vi "Log Pump.vi"(1 "Log File Cluster":T1, 2 "Pumps power":dbl(slide) scale=0.0..100.0 scale format="%#_g%%") -> ()   [LabVIEW 2016]
uses:
  Log File Cluster.ctl
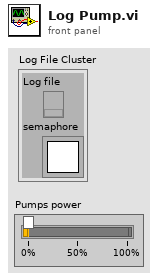
[diagram p1: front panel]
types:
  T1 = typedef "Log File Cluster.ctl" = cluster{"Log file":refnum<k34>, "semaphore":T2}
  T2 = typedef "Semaphore RefNum" = refnum<k1>
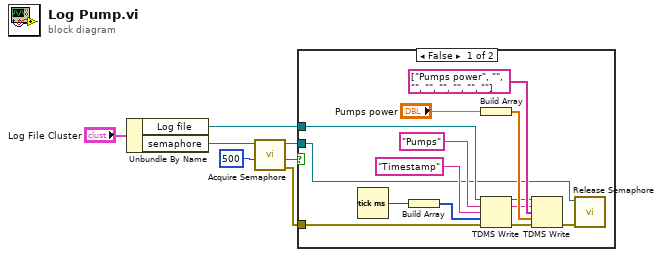
[diagram p0: block diagram]
diagram:
  n1 = Unbundle By Name("Log File Cluster") -> ("Log file"=w6:refnum<k34>, "semaphore"=w5:T2)
  n2 = call <vilib>:"Acquire Semaphore.vi"("ms timeout (-1)"=500, "semaphore"=w5) -> ("error out"=w3:errorcluster, "timed out"=w1:bool, "semaphore out"=w2:T2)  [unwired: 3 in]
  n3 = case shown="False" w1 {
    tunnel: w6 -> [w17 _]
    tunnel: w3 -> [w13 _]
    tunnel: w2 -> [w12 _]
    frame False {
      n4 = Tick Count (ms)() -> (millisecond timer value=w21:u32)
      n5 = Build Array(w21) -> (w20:u32[])
      n6 = Build Array("Pumps power") -> (w14:dbl[])
      n7 = TDMS Write(0:w17, 5:"Pumps" ("group name in (Untitled)"), 7:"Timestamp", 9:w20, 11:w13) -> (4:w9:refnum<k34>, 6:w10:string, 15:w11:errorcluster)  [unwired: 1 in, 1 out]
      n8 = TDMS Write(0:w9, 5:w10, 7:string[] ["Pumps power", "", "", "", "", "", "", ""] ("channel name(s) in (Untitled)"), 9:w14, 11:w11) -> (15:w8:errorcluster)  [unwired: 1 in, 3 out]
      n9 = call <vilib>:"Release Semaphore.vi"("error in (no error)"=w8, "semaphore"=w12) -> ()  [unwired: 4 in, 2 out]
    }
    frame True {
    }
  }
